vi "排气扇监测界面.vi"() -> ()   [LabVIEW 2016, in "环境动力监测库.lvlib"]
uses:
  <vilib>/ptbypt/NI_PtbyPt.lvlib
panel:
  out "排气扇关闭温度":dbl=40.0 caption="关闭温度"
  out "排气扇开启温度":dbl=50.0 caption="开启温度"
  out "输出点":i32
  in  "控制开关":bool
  # "排气扇监测"
  # "℃"
  # "℃"
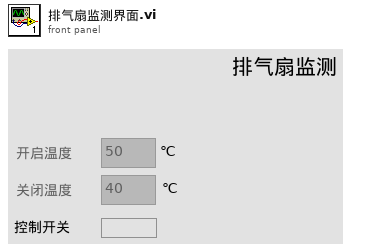
[diagram p1: front panel]
types:
  T1 = cluster{"漏水监测配置":cluster{"监测项描述:输出":string, "端口:":enum16{"AI0", "AI1", "AI2", "AI3", "AI4", "DI0", "DI1", "DI2", "DI3", "DI4", "DO0", "DO1", "DO2", "DO3", "DO4", "X0", "X1", "X2", "X3", "X4", "X5", "X6", "X7", "X8", "X9", "X10", "X11", "X12", "X13", "X14", "X15", "X16", "X17", "X18", "X19", "X20", "X21", "X22", "X23"}, "告警参数:":enum32{"禁用告警", "闭合告警", "断开告警"}, "传感器型号:":enum16{"PLC", "ZLAN", "ART"}, "声光告警启用":bool}, "门禁开关监测配置":cluster{"监测项描述:输出":string, "端口:":enum16{"AI0", "AI1", "AI2", "AI3", "AI4", "DI0", "DI1", "DI2", "DI3", "DI4", "DO0", "DO1", "DO2", "DO3", "DO4", "X0", "X1", "X2", "X3", "X4", "X5", "X6", "X7", "X8", "X9", "X10", "X11", "X12", "X13", "X14", "X15", "X16", "X17", "X18", "X19", "X20", "X21", "X22", "X23"}, "告警参数:":enum32{"禁用告警", "闭合告警", "断开告警"}, "传感器型号:":enum16{"PLC", "ZLAN", "ART"}, "声光告警启用":bool}, "门禁开关监测配置2":cluster{"监测项描述:输出":string, "端口:":enum16{"AI0", "AI1", "AI2", "AI3", "AI4", "DI0", "DI1", "DI2", "DI3", "DI4", "DO0", "DO1", "DO2", "DO3", "DO4", "X0", "X1", "X2", "X3", "X4", "X5", "X6", "X7", "X8", "X9", "X10", "X11", "X12", "X13", "X14", "X15", "X16", "X17", "X18", "X19", "X20", "X21", "X22", "X23"}, "告警参数:":enum32{"禁用告警", "闭合告警", "断开告警"}, "传感器型号:":enum16{"PLC", "ZLAN", "ART"}, "声光告警启用":bool}, "温湿度监测配置":cluster{"监测项描述:输出":string, "端口:":enum16{"AI0", "AI1", "AI2", "AI3", "AI4", "DI0", "DI1", "DI2", "DI3", "DI4", "DO0", "DO1", "DO2", "DO3", "DO4", "X0", "X1", "X2", "X3", "X4", "X5", "X6", "X7", "X8", "X9", "X10", "X11", "X12", "X13", "X14", "X15", "X16", "X17", "X18", "X19", "X20", "X21", "X22", "X23"}, "告警参数:":enum32{"禁用告警", "闭合告警", "断开告警"}, "传感器型号:":enum16{"PLC", "ZLAN", "ART"}, "声光告警启用":bool}, "烟雾监测配置":cluster{"监测项描述:输出":string, "端口:":enum16{"AI0", "AI1", "AI2", "AI3", "AI4", "DI0", "DI1", "DI2", "DI3", "DI4", "DO0", "DO1", "DO2", "DO3", "DO4", "X0", "X1", "X2", "X3", "X4", "X5", "X6", "X7", "X8", "X9", "X10", "X11", "X12", "X13", "X14", "X15", "X16", "X17", "X18", "X19", "X20", "X21", "X22", "X23"}, "告警参数:":enum32{"禁用告警", "闭合告警", "断开告警"}, "传感器型号:":enum16{"PLC", "ZLAN", "ART"}, "声光告警启用":bool}, "冰箱监测配置":cluster{"监测项描述:输出":string, "端口:":enum16{"AI0", "AI1", "AI2", "AI3", "AI4", "DI0", "DI1", "DI2", "DI3", "DI4", "DO0", "DO1", "DO2", "DO3", "DO4", "X0", "X1", "X2", "X3", "X4", "X5", "X6", "X7", "X8", "X9", "X10", "X11", "X12", "X13", "X14", "X15", "X16", "X17", "X18", "X19", "X20", "X21", "X22", "X23"}, "告警参数:":enum32{"禁用告警", "闭合告警", "断开告警"}, "传感器型号:":enum16{"PLC", "ZLAN", "ART"}, "声光告警启用":bool}, "排气扇监测配置":cluster{"监测项描述:输出":string, "端口:":enum16{"AI0", "AI1", "AI2", "AI3", "AI4", "DI0", "DI1", "DI2", "DI3", "DI4", "DO0", "DO1", "DO2", "DO3", "DO4", "X0", "X1", "X2", "X3", "X4", "X5", "X6", "X7", "X8", "X9", "X10", "X11", "X12", "X13", "X14", "X15", "X16", "X17", "X18", "X19", "X20", "X21", "X22", "X23"}, "告警参数:":enum32{"禁用告警", "闭合告警", "断开告警"}, "传感器型号:":enum16{"PLC", "ZLAN", "ART"}, "声光告警启用":bool}, "红外入侵监测配置":cluster{"监测项描述:输出":string, "端口:":enum16{"AI0", "AI1", "AI2", "AI3", "AI4", "DI0", "DI1", "DI2", "DI3", "DI4", "DO0", "DO1", "DO2", "DO3", "DO4", "X0", "X1", "X2", "X3", "X4", "X5", "X6", "X7", "X8", "X9", "X10", "X11", "X12", "X13", "X14", "X15", "X16", "X17", "X18", "X19", "X20", "X21", "X22", "X23"}, "告警参数:":enum32{"禁用告警", "闭合告警", "断开告警"}, "传感器型号:":enum16{"PLC", "ZLAN", "ART"}, "声光告警启用":bool}, "振动监测配置":cluster{"监测项描述:输出":string, "端口:":enum16{"AI0", "AI1", "AI2", "AI3", "AI4", "DI0", "DI1", "DI2", "DI3", "DI4", "DO0", "DO1", "DO2", "DO3", "DO4", "X0", "X1", "X2", "X3", "X4", "X5", "X6", "X7", "X8", "X9", "X10", "X11", "X12", "X13", "X14", "X15", "X16", "X17", "X18", "X19", "X20", "X21", "X22", "X23"}, "告警参数:":enum32{"禁用告警", "闭合告警", "断开告警"}, "传感器型号:":enum16{"PLC", "ZLAN", "ART"}, "声光告警启用":bool}}
  T2 = cluster{"功能启用":bool, "排气扇开启温度":dbl, "排气扇关闭温度":dbl}
  T3 = cluster{"监测项描述:输出":string, "端口:":enum16{"AI0", "AI1", "AI2", "AI3", "AI4", "DI0", "DI1", "DI2", "DI3", "DI4", "DO0", "DO1", "DO2", "DO3", "DO4", "X0", "X1", "X2", "X3", "X4", "X5", "X6", "X7", "X8", "X9", "X10", "X11", "X12", "X13", "X14", "X15", "X16", "X17", "X18", "X19", "X20", "X21", "X22", "X23"}, "告警参数:":enum32{"禁用告警", "闭合告警", "断开告警"}, "传感器型号:":enum16{"PLC", "ZLAN", "ART"}, "声光告警启用":bool}
  T4 = enum16{"AI0", "AI1", "AI2", "AI3", "AI4", "DI0", "DI1", "DI2", "DI3", "DI4", "DO0", "DO1", "DO2", "DO3", "DO4", "X0", "X1", "X2", "X3", "X4", "X5", "X6", "X7", "X8", "X9", "X10", "X11", "X12", "X13", "X14", "X15", "X16", "X17", "X18", "X19", "X20", "X21", "X22", "X23"}
  T5 = cluster{"状态":cluster{"R0":i16, "R1":i16, "R2":i16, "R3":i16, "R4":i16, "R5":i16, "R6":i16, "R7":i16, "R8":i16, "R9":i16, "R10":i16, "R11":i16, "R12":i16, "R13":i16, "R14":i16, "R15":i16, "R16":i16, "R17":i16, "R18":i16, "R19":i16, "R20":i16, "R21":i16, "R22":i16, "R23":i16, "R24":i16, "R25":i16, "R26":i16, "R27":i16, "R28":i16, "R29":i16, "R30":i16, "R31":i16, "R32":i16, "R33":i16, "R34":i16, "R35":i16, "R36":i16, "R37":i16, "R38":i16, "R39":i16}, "输入状态":bool[], "输出状态":bool[], "参数设置":cluster{"R100":i16, "R101":i16, "R102":i16, "R103":i16, "R104":i16, "R105":i16, "R106":i16, "R107":i16, "R108":i16, "R109":i16, "R110":i16, "R111":i16, "R112":i16, "R113":i16, "R114":i16, "R115":i16, "R116":i16, "R117":i16, "R118":i16, "R119":i16, "R120":i16, "R121":i16, "R122":i16, "R123":i16}, "转换值":cluster{"AD0":sgl, "AD1":sgl, "AD2":sgl, "AD3":sgl, "AD4":sgl, "AD5":sgl}}
  T6 = cluster{"状态":cluster{"R0":i16, "R1":i16, "R2":i16, "R3":i16, "R4":i16, "R5":i16, "R6":i16, "R7":i16, "R8":i16, "R9":i16, "R10":i16, "R11":i16, "R12":i16, "R13":i16, "R14":i16, "R15":i16, "R16":i16, "R17":i16, "R18":i16, "R19":i16, "R20":i16, "R21":i16, "R22":i16, "R23":i16, "R24":i16, "R25":i16, "R26":i16, "R27":i16, "R28":i16, "R29":i16, "R30":i16, "R31":i16, "R32":i16, "R33":i16, "R34":i16, "R35":i16, "R36":i16, "R37":i16, "R38":i16, "R39":i16, "R40":i16, "R41":i16, "R42":i16, "R43":i16, "R44":i16, "R45":i16, "R46":i16, "R47":i16, "R48":i16, "R49":i16, "R50":i16, "R51":i16, "R52":i16, "R53":i16, "R54":i16, "R55":i16, "R56":i16, "R57":i16, "R58":i16, "R59":i16, "R60":i16, "R61":i16, "R62":i16, "R63":i16, "R64":i16, "R65":i16, "R66":i16, "R67":i16, "R68":i16, "R69":i16}, "输入状态":bool[], "输出状态":bool[], "报警簇":bool[], "参数设置":cluster{"R100":i16, "R101":i16, "R102":i16, "R103":i16, "R104":i16, "R105":i16, "R106":i16, "R107":i16, "R108":i16, "R109":i16, "R110":i16, "R111":i16, "R112":i16, "R113":i16, "R114":i16, "R115":i16, "R116":i16, "R117":i16, "R118":i16, "R119":i16, "R120":i16, "R121":i16, "R122":i16, "R123":i16, "R124":i16}, "转换值":cluster{"AD0":sgl, "AD1":sgl, "AD2":sgl, "AD3":sgl, "AD4":sgl, "AD5":sgl}, "看门狗启用":bool, "氨氮模块名称":string, "总磷模块名称":string}
  T7 = cluster{"AD0":dbl, "AD1":dbl, "AD2":dbl, "AD3":dbl, "AD4":dbl, "AD5":dbl, "AD6":dbl, "AD7":dbl}
  T8 = cluster{"温湿度":cluster{"状态":bool, "温度:":sgl, "湿度:":sgl, "详情  ":bool}, "空调":cluster{"状态":bool, "机柜温度:":sgl, "压缩机:":enum16{"停止", "运行"}, "电加热:":enum16{"停止", "运行"}, "详情  ":bool}, "排气扇":cluster{"排气扇":bool, "详情  ":bool}, "冰箱":cluster{"冰箱":bool, "详情  ":bool}}
  T9 = cluster{"环境变量":cluster{"蓄电池电压":dbl, "室温":dbl, "湿度":dbl, "水浸报警":bool, "烟雾报警":bool, "门禁1状态":bool, "门禁2状态":bool}, "ZLAN 6842 MB session":refnum<class "MB_Master.lvclass">, "DI":bool[], "DO":bool[]}
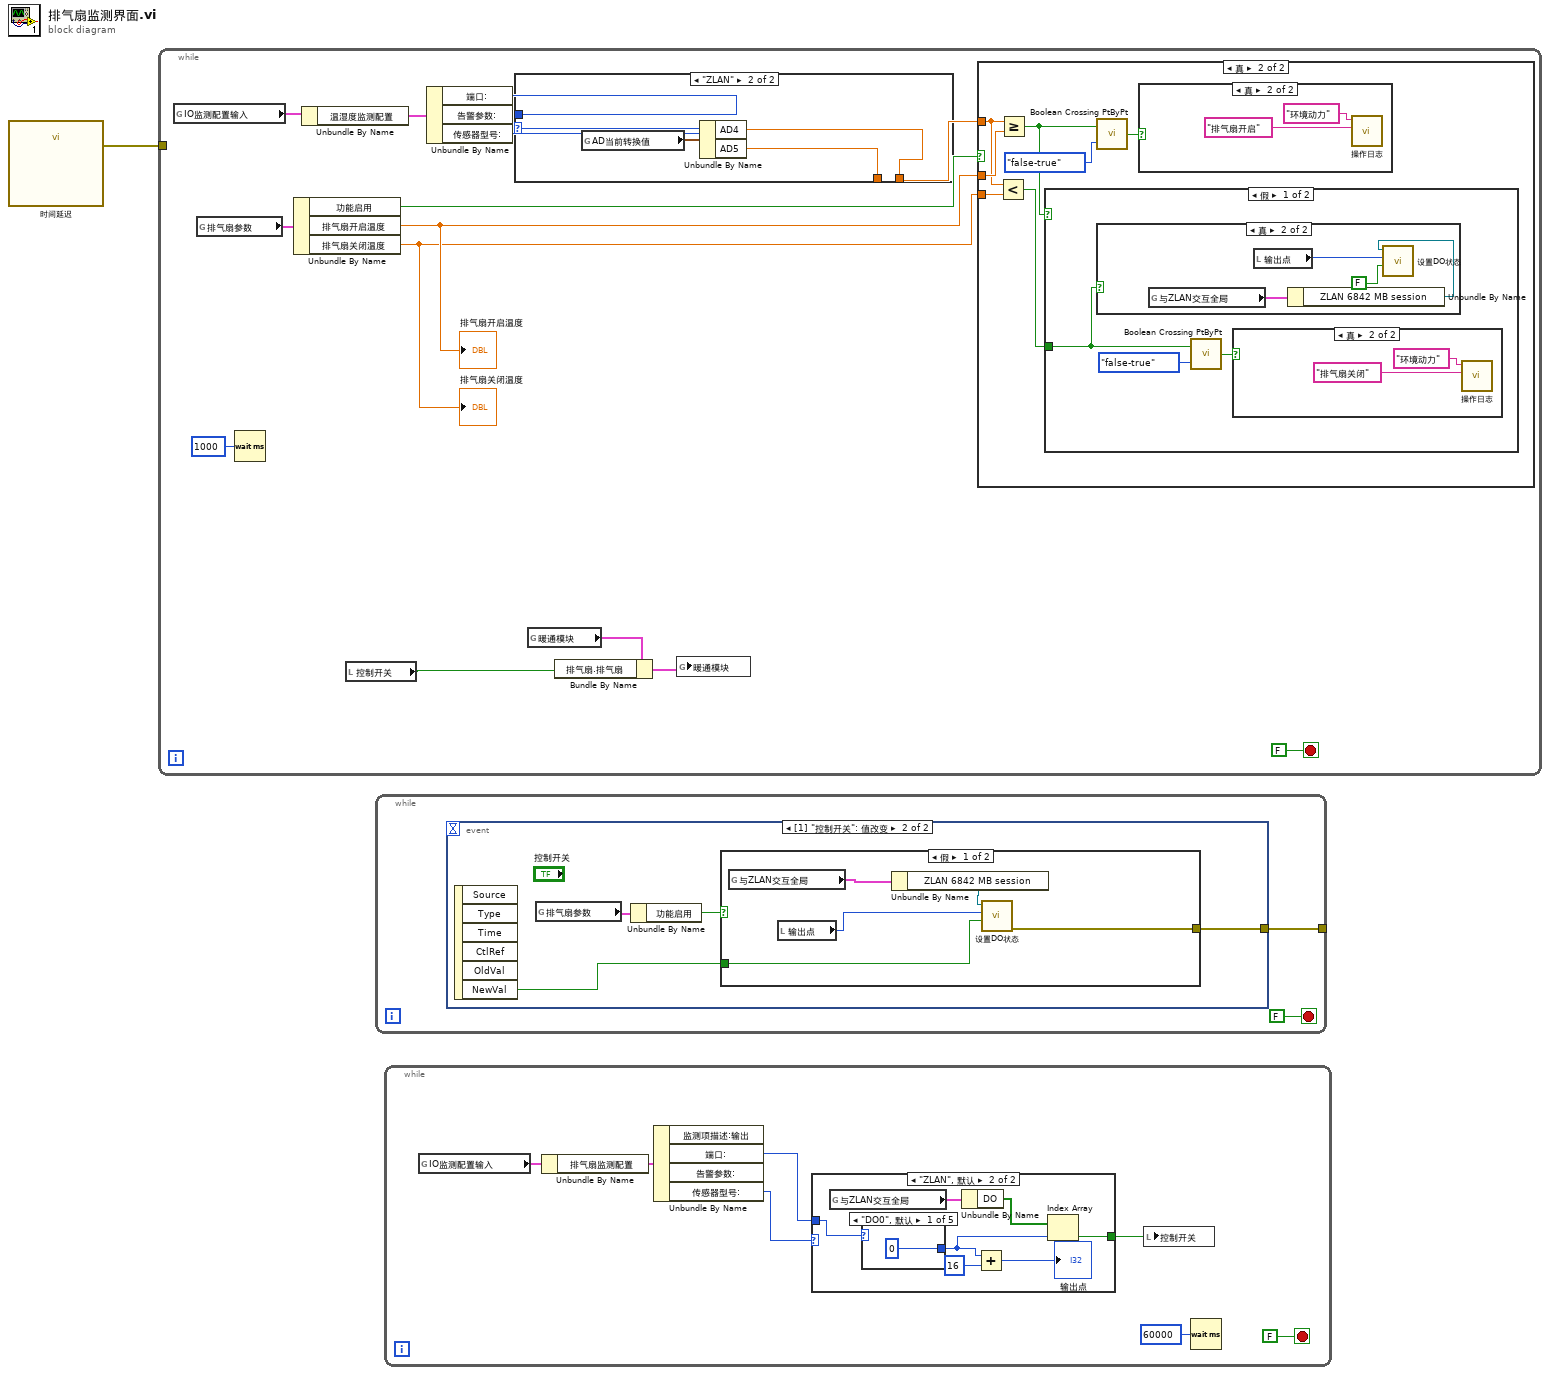
[diagram p0: block diagram]
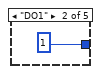
[diagram p3: hidden frame]
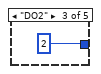
[diagram p4: hidden frame]
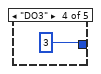
[diagram p5: hidden frame]
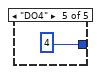
[diagram p6: hidden frame]
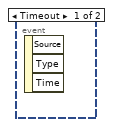
[diagram p7: hidden frame]
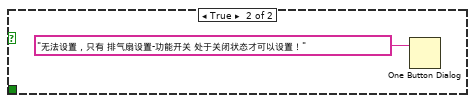
[diagram p8: hidden frame]
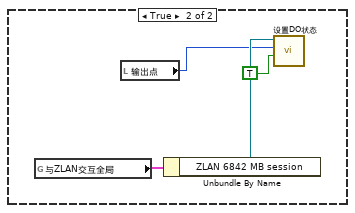
[diagram p13: hidden frame]
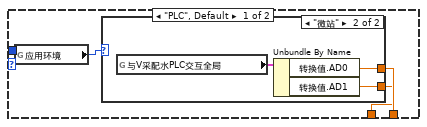
[diagram p14: hidden frame]
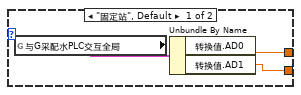
[diagram p15: hidden frame]
diagram:
  n1 = call "时间延迟"() -> ("error out"=w1:errorcluster)  [unwired: 11 in]
  n2 = while {
    tunnel: w1 -> [_]
    stop <- FALSE stop-if-true
    n3 = global read "断电保存全局变量.vi" "IO监测配置输入"() -> (w7:T1)
    n4 = global read "断电保存全局变量.vi" "排气扇参数"() -> (w10:T2)
    n5 = Wait (ms)(milliseconds to wait=u32 1000 ("等待时间（毫秒）")) -> ()  [unwired: 1 out]
    n6 = Unbundle By Name(w10) -> ("功能启用"=w8:bool, "排气扇开启温度"=w3:dbl, "排气扇关闭温度"=w2:dbl)
    "排气扇开启温度" <- w3
    "排气扇关闭温度" <- w2
    n7 = Unbundle By Name(w7) -> ("温湿度监测配置"=w13:T3)
    n8 = local read "控制开关"() -> (w4:bool)
    n9 = Unbundle By Name(w13) -> ("端口:"=w11:T4, "传感器型号:"=w12:enum16{"PLC", "ZLAN", "ART"})  [unwired: 1 out]
    n10 = case shown="\"ZLAN\"" w12 {
      tunnel: w11 -> [_ _]
      tunnel: [w39 w48] -> w9
      tunnel: [w38 w47] -> _
      frame "PLC", Default {
        n11 = global read "外部交互全局变量.vi" "应用环境"() -> (w40:enum16{"固定站", "微站", "浮标", "浮船"})
        n12 = case shown="\"微站\"" w40 {
          tunnel: [w42 w45] -> w39
          tunnel: [w41 w44] -> w38
          frame "固定站", Default {
            n13 = global read "外部交互全局变量.vi" "与G采配水PLC交互全局"() -> (w43:T5)
            n14 = Unbundle By Name(w43) -> ("转换值.AD0"=w42:sgl, "转换值.AD1"=w41:sgl)
          }
          frame "微站" {
            n15 = global read "外部交互全局变量.vi" "与V采配水PLC交互全局"() -> (w46:T6)
            n16 = Unbundle By Name(w46) -> ("转换值.AD0"=w45:sgl, "转换值.AD1"=w44:sgl)
          }
        }
      }
      frame "ZLAN" {
        n17 = global read "断电保存全局变量.vi" "AD当前转换值"() -> (w49:T7)
        n18 = Unbundle By Name(w49) -> ("AD4"=w48:dbl, "AD5"=w47:dbl)
      }
    }
    n19 = global read "内部交互全局变量.vi" "暖通模块"() -> (w6:T8)
    n20 = Bundle By Name(cluster=w6, "排气扇.排气扇"=w4) -> (w5:T8)
    n21 = global write "内部交互全局变量.vi" "暖通模块"(w5) -> ()
    n22 = case shown="真" w8 {
      tunnel: w3 -> [_ w18]
      tunnel: w2 -> [_ w17]
      tunnel: w9 -> [_ w16]
      frame False {
      }
      frame True {
        n23 = Less?(x=w16, y=w17) -> (x < y?=w22:bool)
        n24 = Greater Or Equal?(x=w16, y=w18) -> (x >= y?=w21:bool)
        n25 = case shown="假" w21 {
          tunnel: w22 -> [w25 _]
          frame False {
            n26 = case shown="真" w25 {
              frame False {
              }
              frame True {
                n27 = global read "外部交互全局变量.vi" "与ZLAN交互全局"() -> (w32:T9)
                n28 = local read "输出点"() -> (w30:i32)
                n29 = Unbundle By Name(w32) -> ("ZLAN 6842 MB session"=w31:refnum<class "MB_Master.lvclass">)
                n30 = call "设置DO状态.vi"("value"=FALSE, "address"=w30, "MB session in"=w31) -> ()  [unwired: 7 in, 2 out]
              }
            }
            n31 = call <vilib>:"Boolean Crossing PtByPt.vi"("direction"=enum16{"either", "false-true", "true-false"}."false-true", "input"=w25) -> ("crossing"=w26:bool)  [unwired: 1 in]
            n32 = case shown="真" w26 {
              frame False {
              }
              frame True {
                n33 = call "操作日志.vi"("日志信息"="排气扇关闭", "设备"="环境动力") -> ()  [unwired: 9 in, 1 out]
              }
            }
          }
          frame True {
            n34 = global read "外部交互全局变量.vi" "与ZLAN交互全局"() -> (w36:T9)
            n35 = local read "输出点"() -> (w34:i32)
            n36 = Unbundle By Name(w36) -> ("ZLAN 6842 MB session"=w35:refnum<class "MB_Master.lvclass">)
            n37 = call "设置DO状态.vi"("value"=TRUE, "address"=w34, "MB session in"=w35) -> ()  [unwired: 7 in, 2 out]
          }
        }
        n38 = call <vilib>:"Boolean Crossing PtByPt.vi"("direction"=enum16{"either", "false-true", "true-false"}."false-true", "input"=w21) -> ("crossing"=w20:bool)  [unwired: 1 in]
        n39 = case shown="真" w20 {
          frame False {
          }
          frame True {
            n40 = call "操作日志.vi"("日志信息"="排气扇开启", "设备"="环境动力") -> ()  [unwired: 9 in, 1 out]
          }
        }
      }
    }
  }
  n41 = while {
    tunnel: [w50] -> _
    stop <- FALSE stop-if-true
    n42 = event shown="[1] \"控制开关\": 值改变" {
      selector: _ -> [_ _]
      dyn-events: _ -> [_ _]
      timeout: _ -> [_ _]
      tunnel: [_ w52] -> w50
      event Timeout {
        n43 = event-data() -> ()  [unwired: 1 in, 3 out]
      }
      event "控制开关": Value Change {
        n44 = event-data() -> ("NewVal"=w53:bool)  [unwired: 1 in, 5 out]
        n45 = global read "断电保存全局变量.vi" "排气扇参数"() -> (w55:T2)
        n46 = Unbundle By Name(w55) -> ("功能启用"=w54:bool)
        n47 = case shown="假" w54 {
          tunnel: w53 -> [w60 _]
          tunnel: [w59 _] -> w52
          frame False {
            n48 = global read "外部交互全局变量.vi" "与ZLAN交互全局"() -> (w58:T9)
            n49 = local read "输出点"() -> (w56:i32)
            n50 = Unbundle By Name(w58) -> ("ZLAN 6842 MB session"=w57:refnum<class "MB_Master.lvclass">)
            n51 = call "设置DO状态.vi"("value"=w60, "address"=w56, "MB session in"=w57) -> ("error out"=w59:errorcluster)  [unwired: 7 in, 1 out]
          }
          frame True {
            n52 = One Button Dialog(message="无法设置，只有 排气扇设置-功能开关 处于关闭状态才可以设置！" ("消息")) -> ()  [unwired: 1 in, 1 out]
          }
        }
      }
    }
  }
  n53 = while {
    stop <- FALSE stop-if-true
    n54 = global read "断电保存全局变量.vi" "IO监测配置输入"() -> (w62:T1)
    n55 = Unbundle By Name(w62) -> ("排气扇监测配置"=w66:T3)
    n56 = Unbundle By Name(w66) -> ("端口:"=w64:T4, "传感器型号:"=w65:enum16{"PLC", "ZLAN", "ART"})  [unwired: 2 out]
    n57 = case shown="\"ZLAN\", 默认" w65 {
      tunnel: w64 -> [_ w75]
      tunnel: [_ w74] -> w63
      frame "PLC" {
      }
      frame "ZLAN", Default {
        n58 = global read "外部交互全局变量.vi" "与ZLAN交互全局"() -> (w73:T9)
        n59 = case shown="\"DO0\", 默认" w75 {
          tunnel: [0 1 2 3 4] -> w69
          frame "DO0", Default {
          }
          frame "DO1" {
          }
          frame "DO2" {
          }
          frame "DO3" {
          }
          frame "DO4" {
          }
        }
        n60 = Unbundle By Name(w73) -> ("DO"=w72:bool[])
        n61 = Add(x=w69, y=16) -> (x+y=→"输出点":i32)
        n62 = Index Array(array=w72, index=w69) -> (element=w74:bool)
      }
    }
    n63 = local write "控制开关"(w63) -> ()
    n64 = Wait (ms)(milliseconds to wait=u32 60000 ("等待时间（毫秒）")) -> ()  [unwired: 1 out]
  }
